vi "Obtener Path.vi"(11 "USD Actor.lvlib:USD Actor.lvclass":refnum<class "USD Actor.lvclass">) -> (3 "appended path":path)   [LabVIEW 2019, in "USD Actor.lvlib" / "USD Actor.lvclass"]
uses:
  USD Actor.lvclass
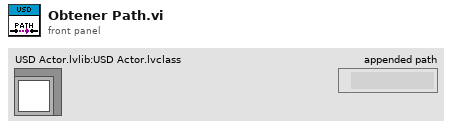
[diagram p1: front panel]
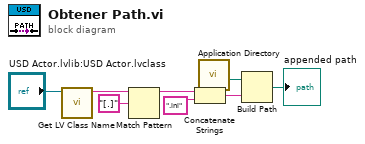
[diagram p0: block diagram]
diagram:
  n1 = call <vilib>:"Get LV Class Name.vi"("object"="USD Actor.lvlib:USD Actor.lvclass") -> ("class name"=w5:string)  [unwired: 9 in, 1 out]
  n2 = Match Pattern(string=w5, regular expression="[.]") -> (before substring=w7:string)  [unwired: 1 in, 3 out]
  n3 = Concatenate Strings(w7, ".ini" ("string")) -> (w8:string)
  n4 = call <vilib>:"Application Directory.vi"() -> ("Application Directory"=w3:path)
  n5 = Build Path(base path=w3, name or relative path=w8) -> (appended path=→"appended path":path)
